vi "packet Handler.vi"   [LabVIEW 2016, in "dxl_x86_c.lvlib"]
doc: "WINDECLSPEC void packetHandler ();"
uses:
  dxl_x86_c.lvlib
  dxl_x86_c.dll
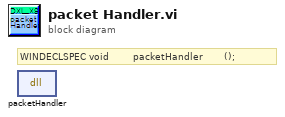
[diagram p0: block diagram]
diagram:
  # "WINDECLSPEC void        packetHandler       ();"
  n1 = dll-call lib="C:/Users/Platform/Desktop/DynamixelSDK/labview/dxl_x86_c.lvlib/dxl_x86_c.*" fn="packetHandler"() -> ()  [unwired: 4 in, 2 out]
